vi "libssh2_session_hostkey.vi"(8 "error in (no error)":errorcluster, 11 "session":u64) -> (0 "error out":errorcluster, 2 "type":i32, 3 "return value":u8[](array[numeric]))   [LabVIEW 2013, in "libssh2.lvlib"]
uses:
  libssh2.lvlib
  libssh2.dll
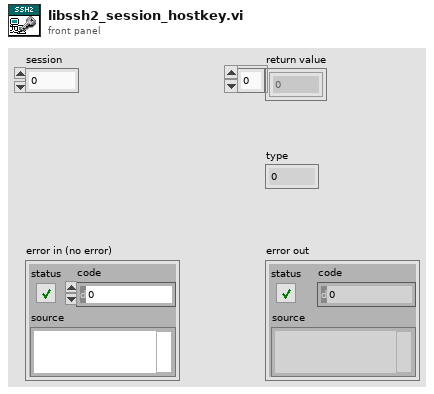
[diagram p1: front panel]
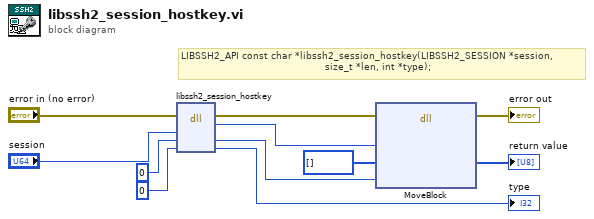
[diagram p0: block diagram]
diagram:
  # "LIBSSH2_API const char *libssh2_session_hostkey(LIBSSH2_SESSION *session,\n                                                size_t *len, int *type);"
  n1 = dll-call lib="C:/Users/pasca/source/repos/libssh2-labview/libssh2**.*" fn="libssh2_session_hostkey"(error in="error in (no error)", "session"="session", "len"=i64 0, "type"=0) -> (error out=w5:errorcluster, "return value"=w6:u64, "len"=w1:i64, "type"=→"type":i32)  [unwired: 3 in, 1 out]
  n2 = dll-call lib="LabVIEW" fn="MoveBlock"(error in=w5, "ps"=w6, "pd"=u8[] [], "size"=w1) -> (error out=→"error out":errorcluster, "pd"=→"return value":u8[])  [unwired: 5 in, 1 out]
